vi "运维调试.vi"() -> ()   [LabVIEW 2016]
uses:
  <vilib>/Utility/miscctls.llb/LVPointTypeDef.ctl
  PLC/PLC.lvlib
  <vilib>/Utility/config.llb/NI_LVConfig.lvlib
panel:
  in  "运维调试菜单":T1(xcontrol)
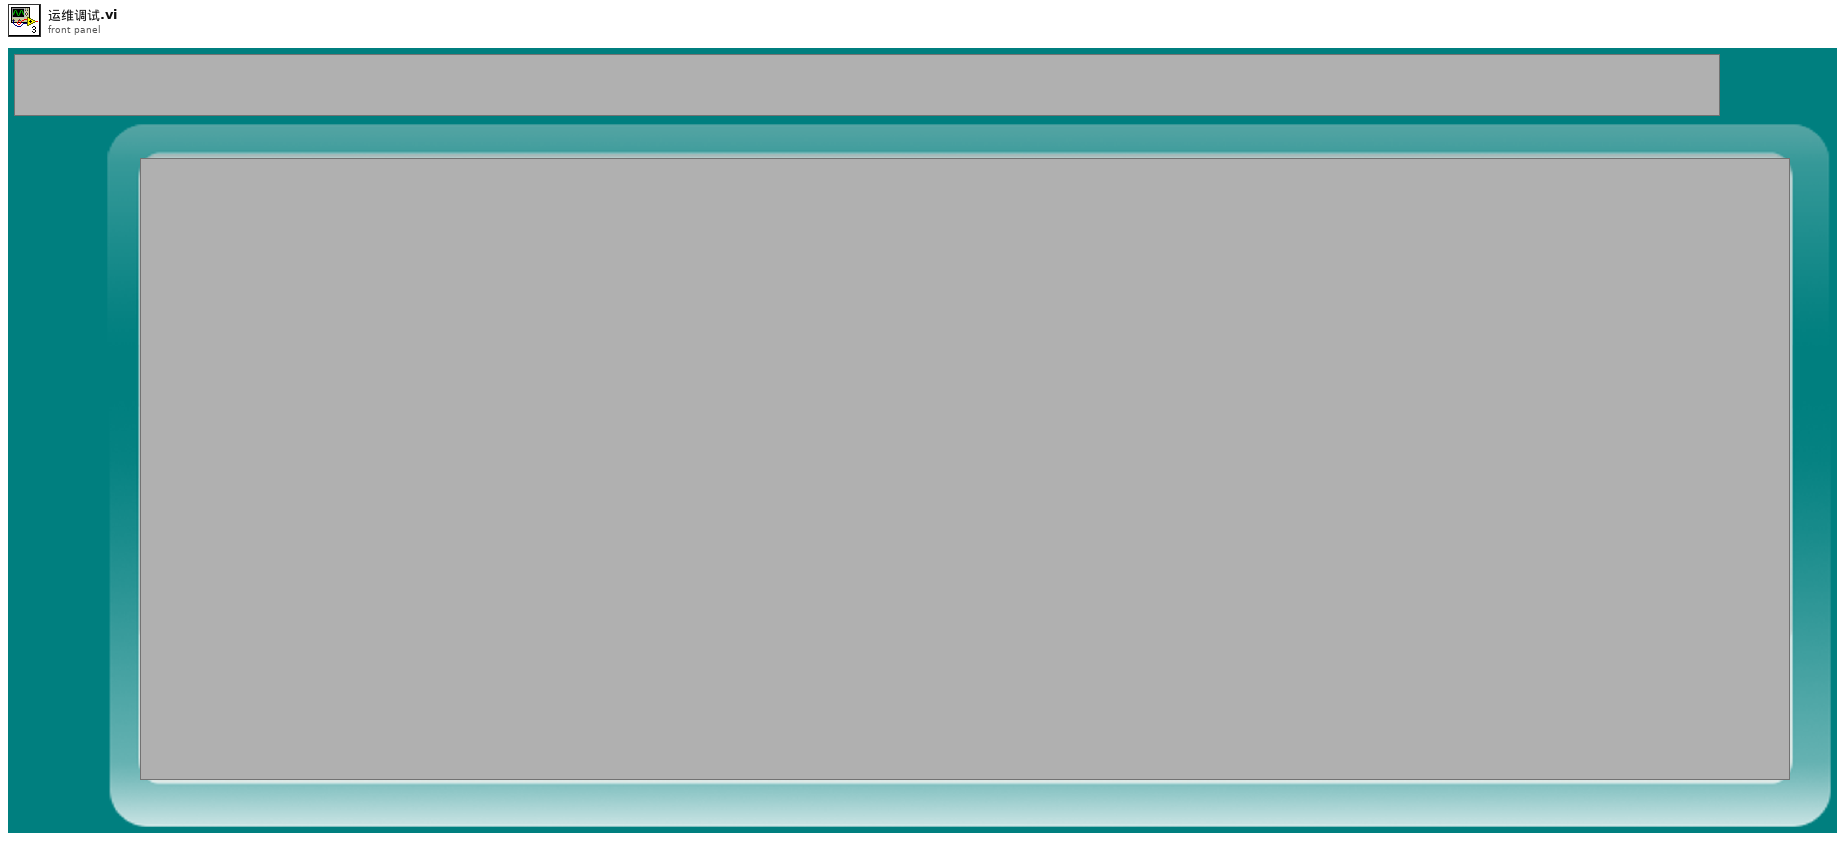
[diagram p1: front panel]
types:
  T1 = enum16{"电源管理", "采配水", "氨氮", "总磷总氮", "多参数", "CODMn", "CODcr", "流量计", "质控单元", "其他"}
  T2 = typedef "NI_LVConfig.lvlib/Config Data RefNum.ctl" = refnum<k1>
  T3 = typedef "LVPointTypeDef.ctl" = cluster{"Horizontal":i16, "Vertical":i16}
  T4 = enum16{"Enabled", "Disabled", "Disabled and Grayed Out"}
  T5 = enum32{"Bad", "Idle", "Run top level", "Running"}
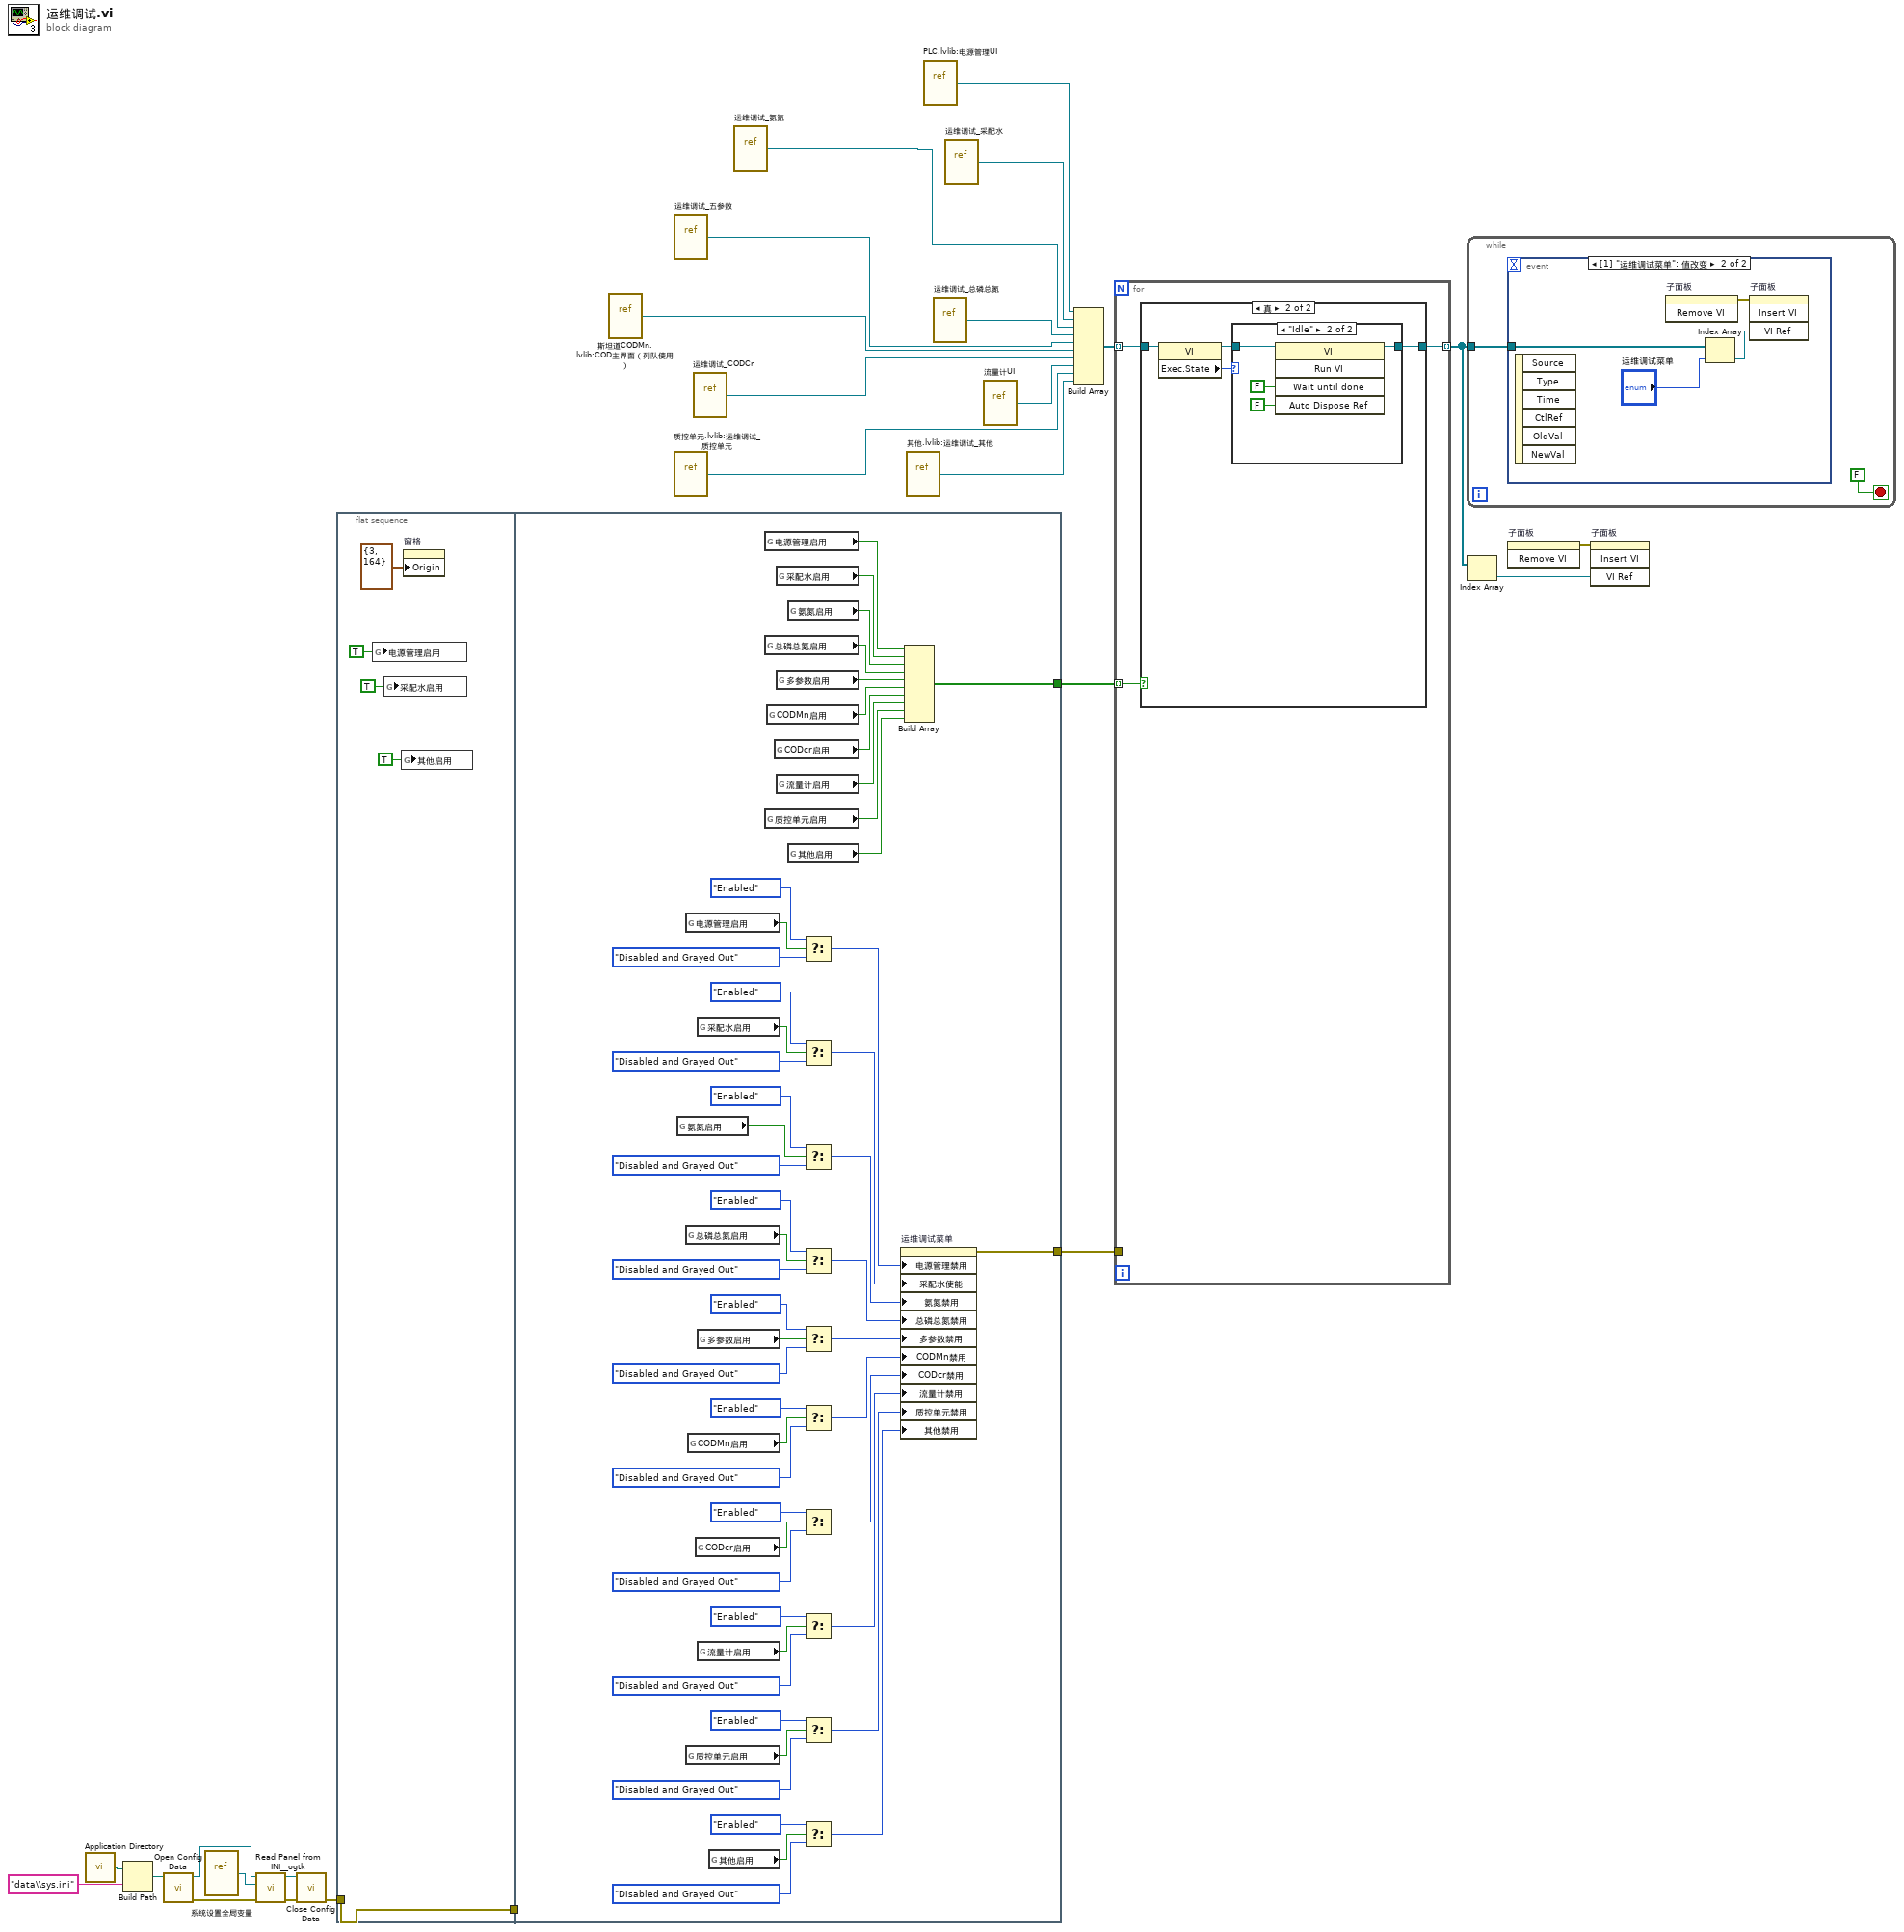
[diagram p0: block diagram]
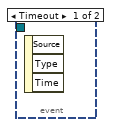
[diagram p4: hidden frame]
diagram:
  n1 = call <vilib>:"Application Directory.vi"() -> ("Application Directory"=w5:path)
  n2 = Build Path(base path=w5, name or relative path="data\\sys.ini" ("名称或相对路径")) -> (appended path=w3:path)
  n3 = call <vilib>:"Open Config Data.vi"("configuration file path"=w3) -> ("error out"=w12:errorcluster, "refnum"=w11:T2)  [unwired: 8 in, 1 out]
  n4 = vi-ref "系统设置全局变量.vi"() -> (w10:refnum<vi>)
  n5 = call <userlib>:"Read Panel from INI__ogtk.vi"("error in (no error)"=w12, "VI ref"=w10, "refnum"=w11) -> ("error out"=w9:errorcluster, "refnum out"=w8:T2)  [unwired: 7 in]
  n6 = call <vilib>:"Close Config Data.vi"("error in (no error)"=w9, "refnum"=w8) -> ("error out"=w7:errorcluster)  [unwired: 8 in, 1 out]
  n7 = flat-sequence {
    tunnel: w7 -> [w31]
    tunnel: [w31] -> w6
    tunnel: [w64] -> w13
    tunnel: w6 -> [_]
    tunnel: [w53] -> w2
    frame #0 {
      n8 = global write "系统设置全局变量.vi" "电源管理启用"(TRUE ("电源管理启用")) -> ()
      n9 = global write "系统设置全局变量.vi" "采配水启用"(TRUE ("采配水启用")) -> ()
      n10 = global write "系统设置全局变量.vi" "其他启用"(TRUE ("其他启用")) -> ()
      n11 = property on="窗格" class="Pane"("Origin"=T3 {"Horizontal"=3, "Vertical"=164} ("原点")) -> ()  [unwired: 2 in, 2 out]
    }
    frame #1 {
      n12 = global read "系统设置全局变量.vi" "氨氮启用"() -> (w32:bool)
      n13 = global read "系统设置全局变量.vi" "电源管理启用"() -> (w83:bool)
      n14 = global read "系统设置全局变量.vi" "总磷总氮启用"() -> (w78:bool)
      n15 = global read "系统设置全局变量.vi" "质控单元启用"() -> (w71:bool)
      n16 = global read "系统设置全局变量.vi" "CODMn启用"() -> (w74:bool)
      n17 = global read "系统设置全局变量.vi" "CODcr启用"() -> (w73:bool)
      n18 = global read "系统设置全局变量.vi" "采配水启用"() -> (w80:bool)
      n19 = global read "系统设置全局变量.vi" "多参数启用"() -> (w76:bool)
      n20 = global read "系统设置全局变量.vi" "流量计启用"() -> (w72:bool)
      n21 = global read "系统设置全局变量.vi" "其他启用"() -> (w70:bool)
      n22 = global read "系统设置全局变量.vi" "电源管理启用"() -> (w54:bool)
      n23 = global read "系统设置全局变量.vi" "总磷总氮启用"() -> (w57:bool)
      n24 = global read "系统设置全局变量.vi" "质控单元启用"() -> (w62:bool)
      n25 = global read "系统设置全局变量.vi" "CODMn启用"() -> (w59:bool)
      n26 = global read "系统设置全局变量.vi" "CODcr启用"() -> (w60:bool)
      n27 = global read "系统设置全局变量.vi" "采配水启用"() -> (w55:bool)
      n28 = global read "系统设置全局变量.vi" "多参数启用"() -> (w58:bool)
      n29 = global read "系统设置全局变量.vi" "流量计启用"() -> (w61:bool)
      n30 = global read "系统设置全局变量.vi" "氨氮启用"() -> (w56:bool)
      n31 = global read "系统设置全局变量.vi" "其他启用"() -> (w63:bool)
      n32 = Select(t=T4."Enabled" ("电源管理禁用"), s=w83, f=T4."Disabled and Grayed Out" ("电源管理禁用")) -> (s? t:f=w82:T4)
      n33 = Select(t=T4."Enabled" ("电源管理禁用"), s=w80, f=T4."Disabled and Grayed Out" ("电源管理禁用")) -> (s? t:f=w81:T4)
      n34 = Select(t=T4."Enabled" ("电源管理禁用"), s=w32, f=T4."Disabled and Grayed Out" ("电源管理禁用")) -> (s? t:f=w79:T4)
      n35 = Select(t=T4."Enabled" ("电源管理禁用"), s=w78, f=T4."Disabled and Grayed Out" ("电源管理禁用")) -> (s? t:f=w77:T4)
      n36 = Select(t=T4."Enabled" ("电源管理禁用"), s=w76, f=T4."Disabled and Grayed Out" ("电源管理禁用")) -> (s? t:f=w75:T4)
      n37 = Select(t=T4."Enabled" ("电源管理禁用"), s=w74, f=T4."Disabled and Grayed Out" ("电源管理禁用")) -> (s? t:f=w69:T4)
      n38 = Select(t=T4."Enabled" ("电源管理禁用"), s=w73, f=T4."Disabled and Grayed Out" ("电源管理禁用")) -> (s? t:f=w68:T4)
      n39 = Select(t=T4."Enabled" ("电源管理禁用"), s=w72, f=T4."Disabled and Grayed Out" ("电源管理禁用")) -> (s? t:f=w67:T4)
      n40 = Select(t=T4."Enabled" ("电源管理禁用"), s=w71, f=T4."Disabled and Grayed Out" ("电源管理禁用")) -> (s? t:f=w66:T4)
      n41 = Select(t=T4."Enabled" ("电源管理禁用"), s=w70, f=T4."Disabled and Grayed Out" ("电源管理禁用")) -> (s? t:f=w65:T4)
      n42 = property on="运维调试菜单" class="运维调试菜单 (严格)"("电源管理禁用"=w82, "采配水使能"=w81, "氨氮禁用"=w79, "总磷总氮禁用"=w77, "多参数禁用"=w75, "CODMn禁用"=w69, "CODcr禁用"=w68, "流量计禁用"=w67, "质控单元禁用"=w66, "其他禁用"=w65) -> (error out=w64:errorcluster)  [unwired: 2 in, 1 out]
      n43 = Build Array(w54, w55, w56, w57, w58, w59, w60, w61, w62, w63) -> (w53:bool[])
    }
  }
  n44 = vi-ref "斯坦道CODMn.lvlib:COD主界面（列队使用）.vi"() -> (w19:refnum<vi>)
  n45 = vi-ref "运维调试_五参数.vi"() -> (w20:refnum<vi>)
  n46 = vi-ref "质控单元.lvlib:运维调试_质控单元.vi"() -> (w17:refnum<vi>)
  n47 = vi-ref "运维调试_CODCr.vi"() -> (w18:refnum<vi>)
  n48 = vi-ref "运维调试_氨氮.vi"() -> (w1:refnum<vi>)
  n49 = vi-ref "其他.lvlib:运维调试_其他.vi"() -> (w16:refnum<vi>)
  n50 = vi-ref "PLC.lvlib:电源管理UI.vi"() -> (w15:refnum<vi>)
  n51 = vi-ref "运维调试_总磷总氮.vi"() -> (w21:refnum<vi>)
  n52 = vi-ref "运维调试_采配水.vi"() -> (w22:refnum<vi>)
  n53 = vi-ref "流量计UI.vi"() -> (w14:refnum<vi>)
  n54 = Build Array(w15, w22, w1, w21, w20, w19, w18, w14, w17, w16) -> (w23:refnum<vi>[])
  n55 = for {
    tunnel: w23 -> [w86] mode=indexing
    tunnel: [w85] -> w25 mode=indexing
    tunnel: w2 -> [w84] mode=indexing
    tunnel: w13 -> [_]
    n56 = case shown="真" w84 {
      tunnel: w86 -> [w87 w91]
      tunnel: [w87 w88] -> w85
      frame False {
      }
      frame True {
        n57 = property class="VI"(reference=w91) -> (reference out=w89:refnum<vi>, "Exec.State"=w90:T5)  [unwired: 1 in, 1 out]
        n58 = case shown="\"Idle\"" w90 {
          tunnel: w89 -> [w92 w94]
          tunnel: [w92 w93] -> w88
          frame "Bad", Default {
          }
          frame "Idle" {
            n59 = invoke class="VI" method="Run VI"(reference=w94, "Wait until done"=FALSE ("结束前等待"), "Auto Dispose Ref"=FALSE ("自动销毁引用")) -> (reference out=w93:refnum<vi>)  [unwired: 2 in, 4 out]
          }
        }
      }
    }
  }
  n60 = while {
    tunnel: w25 -> [w97]
    stop <- FALSE stop-if-true
    n61 = event shown="[1] \"运维调试菜单\": 值改变" {
      selector: _ -> [_ _]
      dyn-events: _ -> [_ _]
      timeout: _ -> [_ _]
      tunnel: w97 -> [_ w101]
      event Timeout {
        n62 = event-data() -> ()  [unwired: 1 in, 3 out]
      }
      event "运维调试菜单": Value Change {
        n63 = event-data() -> ()  [unwired: 1 in, 6 out]
        n64 = invoke on="子面板" class="SubPnl" method="Remove VI"() -> (error out=w102:errorcluster)  [unwired: 3 in, 2 out]
        n65 = Index Array(array=w101, index="运维调试菜单") -> (element=w100:refnum<vi>)
        n66 = invoke on="子面板" class="SubPnl" method="Insert VI"(error in=w102, "VI Ref"=w100) -> ()  [unwired: 2 in, 4 out]
      }
    }
  }
  n67 = Index Array(array=w25) -> (element=w24:refnum<vi>)  [unwired: 1 in]
  n68 = invoke on="子面板" class="SubPnl" method="Remove VI"() -> (error out=w26:errorcluster)  [unwired: 3 in, 2 out]
  n69 = invoke on="子面板" class="SubPnl" method="Insert VI"(error in=w26, "VI Ref"=w24) -> ()  [unwired: 2 in, 4 out]
